vi "SR430 Getting Started.vi"() -> ()   [LabVIEW 2009, in "SR430Driver.lvlib"]
doc: "\"Getting Started\" and first application example.\n\nCopyright (C)\nGesellschaft für Schwerionenforschung, GSI\nPlanckstr. 1\n64291 Darmstadt\nGermany\n\nContact: D.Beck@gsi.de \n\nThis program is free software; you can redistribute it and/or modify it under the terms of the \nGNU General Public License as published by the Free Software Foundation; either version 2 of the license, or (at your option) any later version.\n\nThis program is distributed in the hope that it will be useful, but WITHOUT ANY WARRANTY; without even the implied warranty of MERCHANTABILITY or FITNESS FOR A PARTICULAR PURPOSE. See the GNU General License for more details (http://www.gnu.org).\n\nGesellschaft für Schwerionenforschung, GSI\nPlanckstr. 1, 64291 Darmstadt, Germany\nFor all questions and ideas contact: M.Richter@gsi.de, K.Poppensieker, H.Brand@gsi.de or D.Beck@gsi.de.\nLast update: 11-APR-2002"
uses:
  SR430Driver.lvlib
  SR430_VISA Control.ctl
panel:
  in  "stop":bool
  out "Waveform Graph":u16[](graph)
  out "data sum":u32
  in  "get data":bool
  in  "start":bool
  in  "bins per record":i32
  in  "records per scan":i32
  in  "bin width":i32
  in  "configure":bool
  in  "init":bool
  in  "cursor on":bool
  in  "discriminator level [V]":dbl=0.2 format="%.2f"
  in  "discriminatorSlope":bool=TRUE
  in  "triggerSlope":bool=TRUE
  in  "trigger level [V]":dbl=1.0 format="%.2f"
  in  "VISA resource":T1={"VISA resource name"="SR430"}
  out "error out":errorcluster
  # "SR430 Getting Started"
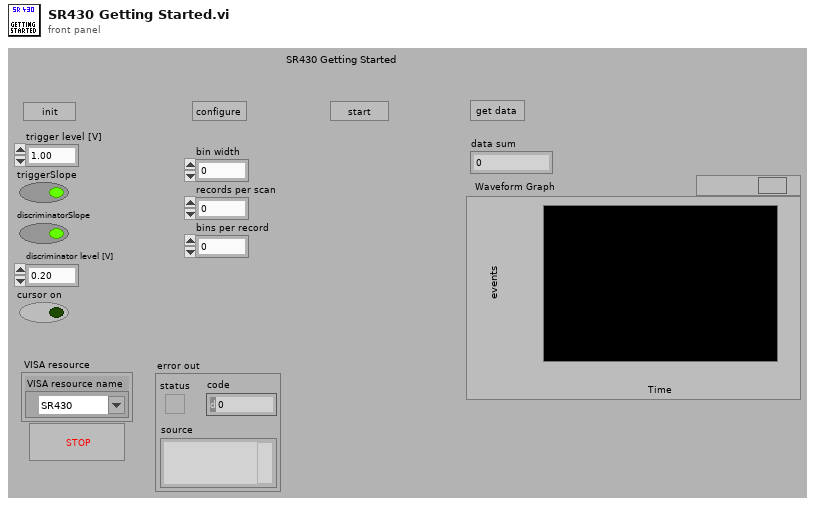
[diagram p1: front panel]
types:
  T1 = typedef "SR430Driver.lvlib/SR430_VISA Control.ctl" = cluster{"VISA resource name":refnum<visa-resource-name>}
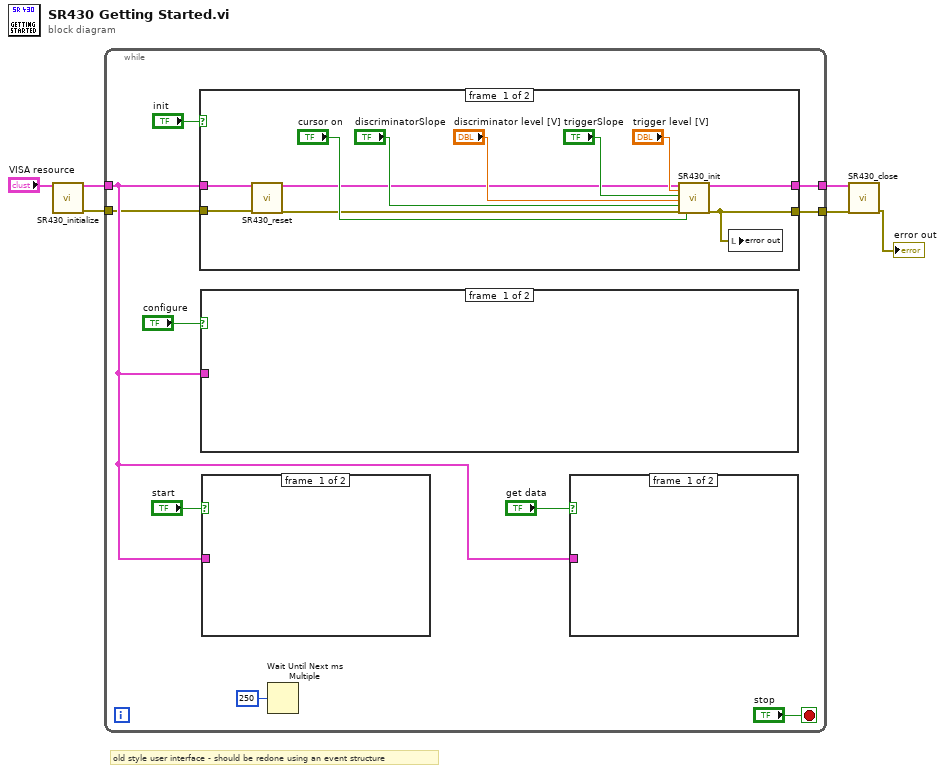
[diagram p0: block diagram]
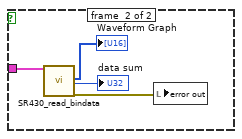
[diagram p2: hidden frame]
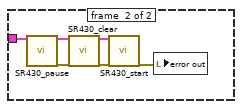
[diagram p3: hidden frame]
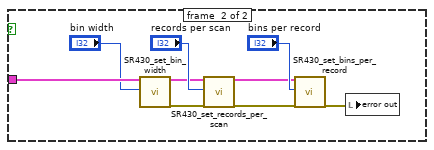
[diagram p4: hidden frame]
diagram:
  # "old style user interface - should be redone using an event structure"
  n1 = call "SR430_initialize.vi"("SR430 VISA Cluster"="VISA resource") -> ("SR430 VISA Cluster out"=w6:T1, "error out"=w2:errorcluster)  [unwired: 11 in, 2 out]
  n2 = while {
    tunnel: w6 -> [w10]
    tunnel: [w9] -> w4
    tunnel: w2 -> [w8]
    tunnel: [w7] -> w1
    stop <- "stop" stop-if-true
    n3 = case shown="True" "init" {
      tunnel: w10 -> [w46 w48]
      tunnel: [w39 w48] -> w9
      tunnel: w8 -> [w38 w47]
      tunnel: [w36 w47] -> w7
      frame #0 {
        n4 = call "SR430_reset.vi"("address"=w46, "error in (no error)"=w38) -> ("address out"=w40:T1, "error out"=w37:errorcluster)  [unwired: 16 in]
        n5 = call "SR430_init.vi"("GPIB address"=w40, "triggeLevel [V]"="trigger level [V]", "triggerSlope"="triggerSlope", "discriminatorLevel [V]"="discriminator level [V]", "discriminatorSlope"="discriminatorSlope", "error in (no error)"=w37, "cursorOn"="cursor on") -> ("GPIB address out"=w39:T1, "error out"=w36:errorcluster)  [unwired: 11 in]
        n6 = local write "error out"(w36) -> ()
      }
      frame #1 {
      }
    }
    n7 = case shown="True" "configure" {
      tunnel: w10 -> [_ w35]
      frame #0 {
      }
      frame #1 {
        n8 = call "SR430_set_bin_width.vi"("address"=w35, "binWidth"="bin width") -> ("address out"=w27:T1, "error out"=w29:errorcluster)  [unwired: 16 in]
        n9 = call "SR430_set_records_per_scan.vi"("address string"=w27, "recordsPerScan"="records per scan", "error in (no error)"=w29) -> ("address out"=w31:T1, "error out"=w30:errorcluster)  [unwired: 15 in]
        n10 = call "SR430_set_bins_per_record.vi"("address"=w31, "binsPerRecord"="bins per record", "error in (no error)"=w30) -> ("error out"=w28:errorcluster)  [unwired: 15 in, 1 out]
        n11 = local write "error out"(w28) -> ()
      }
    }
    n12 = case shown="True" "start" {
      tunnel: w10 -> [_ w22]
      frame #0 {
      }
      frame #1 {
        n13 = call "SR430_pause.vi"("address"=w22) -> ("address out"=w21:T1, "error out"=w23:errorcluster)  [unwired: 17 in]
        n14 = call "SR430_clear.vi"("address"=w21, "error in (no error)"=w23) -> ("address out"=w26:T1, "error out"=w25:errorcluster)  [unwired: 16 in]
        n15 = call "SR430_start.vi"("address"=w26, "error in (no error)"=w25) -> ("error out"=w24:errorcluster)  [unwired: 16 in, 1 out]
        n16 = local write "error out"(w24) -> ()
      }
    }
    n17 = Wait Until Next ms Multiple(millisecond multiple=u32 250) -> ()  [unwired: 1 out]
    n18 = case shown="True" "get data" {
      tunnel: w10 -> [_ w20]
      frame #0 {
      }
      frame #1 {
        n19 = call "SR430_read_bindata.vi"("address"=w20) -> ("Data"=→"Waveform Graph":u16[], "dataSum"=→"data sum":u32, "error out"=w19:errorcluster)  [unwired: 15 in, 1 out]
        n20 = local write "error out"(w19) -> ()
      }
    }
  }
  n21 = call "SR430_close.vi"("SR430 VISA Cluster"=w4, "error in (no error)"=w1) -> ("error out"=→"error out":errorcluster)  [unwired: 13 in]
